vi "cw_4_5.vi"() -> ()   [LabVIEW 2022 SP3]
panel:
  out "result string":string
  in  "Input":string
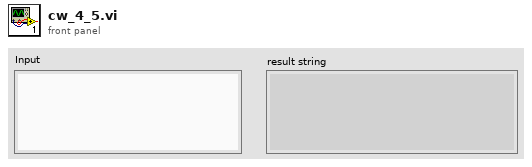
[diagram p1: front panel]
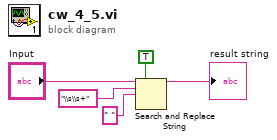
[diagram p0: block diagram]
diagram:
  n1 = Search and Replace String(replace all?=TRUE ("replace all? (F)"), input string="Input", search string="\\s\\s+" ("regular expression"), replace string=" " ("replace string (\"\")")) -> (result string=→"result string":string)  [unwired: 4 in, 3 out]
